vi "Device Test Suite.vi"() -> ()   [LabVIEW 2018]
panel:
  out "Status":T1
  in  "Test":bool
  in  "stop":bool
  in  "Function":u16(ring) items=["Set position", "Get position", "Get status", "Other settings"]
  out "Position out":dbl[](array[numeric])
  in  "Position in":dbl[](array[numeric])
  in  "vi path":path
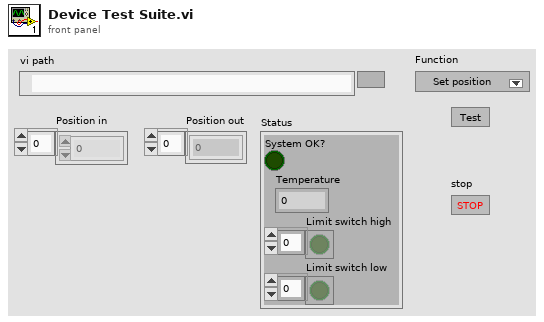
[diagram p1: front panel]
types:
  T1 = cluster{"System OK?":bool, "Temperature":dbl, "Limit switch high":bool[], "Limit switch low":bool[]}
  T2 = enum16{"Initialize", "Shut down", "Set position", "Get position", "Get status", "Other settings"}
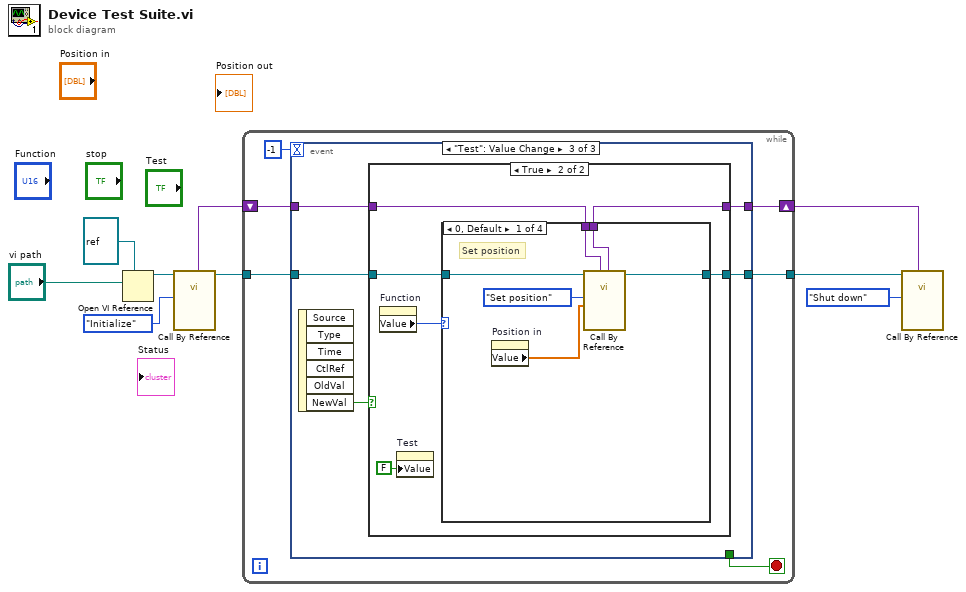
[diagram p0: block diagram]
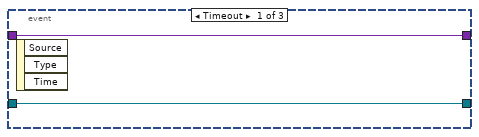
[diagram p2: hidden frame]
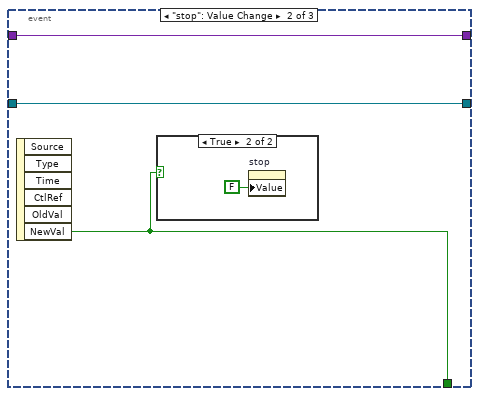
[diagram p3: hidden frame]
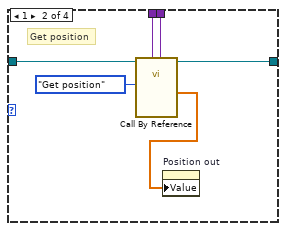
[diagram p6: hidden frame]
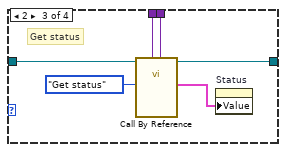
[diagram p7: hidden frame]
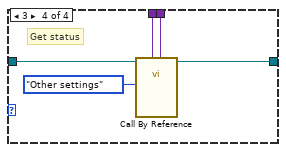
[diagram p8: hidden frame]
diagram:
  n1 = Open VI Reference(type specifier VI Refnum (for type only)=refnum<vi> refnum, vi path="vi path") -> (vi reference=w8:refnum<vi>)  [unwired: 4 in, 1 out]
  n2 = call-by-ref "?"(reference=w8, "Operation"=T2."Initialize") -> (reference out=w5:refnum<vi>, "Device-specific out"=w2:variant)  [unwired: 7 in, 5 out]
  n3 = while {
    tunnel: [w14] -> w4
    tunnel: w5 -> [w13]
    shift-right: [w10] -> w1
    shift-left: w2 -> [w11]
    stop <- w15 stop-if-true
    n4 = event shown="[2] \"Test\": Value Change" {
      selector: _ -> [_ _ _]
      dyn-events: _ -> [_ _ _]
      timeout: -1 -> [_ _ _]
      tunnel: [_ w19 _] -> w15
      tunnel: [w17 w20 w24] -> w14
      tunnel: w13 -> [w17 w20 w25]
      tunnel: w11 -> [w16 w18 w23]
      tunnel: [w16 w18 w22] -> w10
      event Timeout {
        n5 = event-data() -> ()  [unwired: 1 in, 3 out]
      }
      event "stop": Value Change {
        n6 = event-data() -> ("NewVal"=w19:bool)  [unwired: 1 in, 5 out]
        n7 = case shown="True" w19 {
          frame False {
          }
          frame True {
            n8 = property on="stop" class="Bool (strict)"("Value"=FALSE ("stop")) -> ()  [unwired: 2 in, 2 out]
          }
        }
      }
      event "Test": Value Change {
        n9 = event-data() -> ("NewVal"=w26:bool)  [unwired: 1 in, 5 out]
        n10 = case shown="True" w26 {
          tunnel: w25 -> [w28 w33]
          tunnel: [w28 w32] -> w24
          tunnel: w23 -> [w27 w30]
          tunnel: [w27 w29] -> w22
          frame False {
          }
          frame True {
            n11 = property on="Function" class="Ring (strict)"() -> ("Value"=w31:u16)  [unwired: 2 in, 2 out]
            n12 = property on="Test" class="Bool (strict)"("Value"=FALSE ("Test")) -> ()  [unwired: 2 in, 2 out]
            n13 = case shown="0, Default" w31 {
              tunnel: w33 -> [w40 w46 w52 w57]
              tunnel: [w39 w45 w51 w56] -> w32
              tunnel: w30 -> [w36 w42 w48 w54]
              tunnel: [w35 w41 w47 w53] -> w29
              frame 0, Default {
                # "Set position"
                n14 = property on="Position in" class="Arr (strict)"() -> ("Value"=w37:dbl[])  [unwired: 2 in, 2 out]
                n15 = call-by-ref "?"(reference=w40, "Device-specific in"=w36, "Position in"=w37, "Operation"=T2."Set position") -> (reference out=w39:refnum<vi>, "Device-specific out"=w35:variant)  [unwired: 5 in, 5 out]
              }
              frame 1 {
                # "Get position"
                n16 = call-by-ref "?"(reference=w46, "Device-specific in"=w42, "Operation"=T2."Get position") -> (reference out=w45:refnum<vi>, "Position out"=w43:dbl[], "Device-specific out"=w41:variant)  [unwired: 6 in, 4 out]
                n17 = property on="Position out" class="Arr (strict)"("Value"=w43) -> ()  [unwired: 2 in, 2 out]
              }
              frame 2 {
                # "Get status"
                n18 = call-by-ref "?"(reference=w52, "Device-specific in"=w48, "Operation"=T2."Get status") -> (reference out=w51:refnum<vi>, "Status"=w49:T1, "Device-specific out"=w47:variant)  [unwired: 6 in, 4 out]
                n19 = property on="Status" class="Clust (strict)"("Value"=w49) -> ()  [unwired: 2 in, 2 out]
              }
              frame 3 {
                # "Get status"
                n20 = call-by-ref "?"(reference=w57, "Device-specific in"=w54, "Operation"=T2."Other settings") -> (reference out=w56:refnum<vi>, "Device-specific out"=w53:variant)  [unwired: 6 in, 5 out]
              }
            }
          }
        }
      }
    }
  }
  n21 = call-by-ref "?"(reference=w4, "Device-specific in"=w1, "Operation"=T2."Shut down") -> ()  [unwired: 6 in, 7 out]
